vi "Write configuration.vi"(8 "error in (no error)":errorcluster, 11 "wavefront sensor in":refnum<class "wavefront sensor.lvclass">) -> (0 "error out":errorcluster, 3 "wavefront sensor out":refnum<class "wavefront sensor.lvclass">)   [LabVIEW 2012, in "wavefront sensor.lvclass"]
doc: "Writes the configuration cluster into the configuration file. Configuration file is XML-based. It's name is <component ID>.xml"
uses:
  wavefront sensor.lvclass
  <vilib>/Distrio/Murmex/Murmex/Murmex.lvclass
  wavefront sensor.lvclass/wavefront sensor.ctl
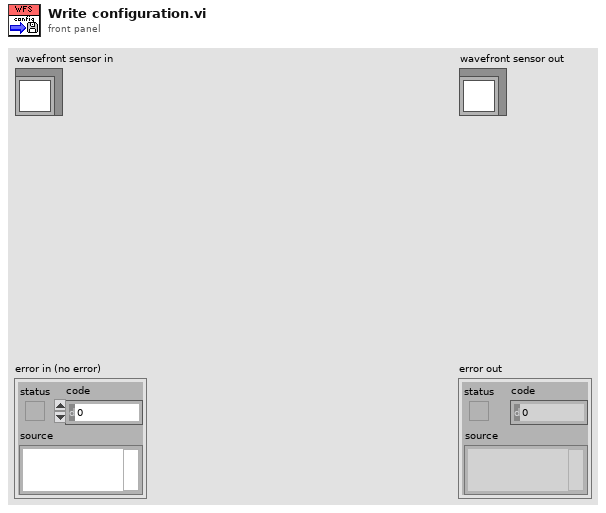
[diagram p1: front panel]
types:
  T1 = typedef "wavefront sensor.lvclass/configuration.ctl" = cluster{"Numeric":dbl}
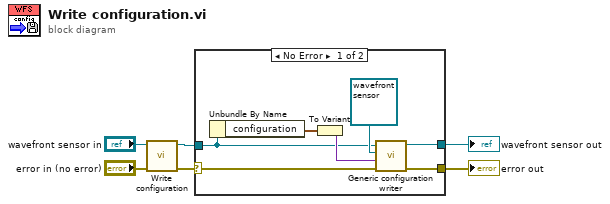
[diagram p0: block diagram]
diagram:
  n1 = call-parent "Write configuration.vi"("error in (no error)"="error in (no error)", "Murmex in"="wavefront sensor in") -> ("error out"=w4:errorcluster, "Murmex out"=w1:refnum<class "wavefront sensor.lvclass">)  [unwired: 8 in]
  n2 = case shown="No Error" w4 {
    selector: w4 -> [w11 w14]
    tunnel: [w10 w14] -> w3
    tunnel: [w9 w15] -> w2
    tunnel: w1 -> [w7 w15]
    frame No Error {
      n3 = Unbundle By Name(w7) -> ("configuration"=w12:T1)
      n4 = To Variant(anything=w12) -> (Variant=w13:variant)
      n5 = call <vilib>:"Generic configuration writer.vi"("error in (no error)"=w11, "configuration"=w13, "inheritance level"=refnum<class "wavefront sensor.lvclass"> refnum ("wavefront sensor"), "MurmexBase in"=w7) -> ("error out"=w10:errorcluster, "MurmexBase out"=w9:refnum<class "wavefront sensor.lvclass">)  [unwired: 6 in]
    }
    frame Error {
    }
  }
  "error out" <- w3
  "wavefront sensor out" <- w2
